vi "BRig_RT__Case_Exp__State_initTrial2.vi"(0 "input_dataCurrent":u16[](array[numeric]), 1 "input_dataTrial":u16[][](array[numeric]), 3 "input_dataExp":u16[](array[numeric]), 6 "input_dataBlock":u16[][](array[numeric]), 8 "input_dataLC":u16[](array[numeric])) -> (7 "output_L_Wrong_Laser_l2":bool, 9 "output_L_Wrong_Event_l2":bool, 10 "output_L_Power_l1":dbl, 11 "output_L_Reward_Laser_l2":bool, 12 "output_L_Power_l2":dbl, 13 "output_L_Reward_Event_l2":bool, 14 "output_dataCurrent":u16[](array[numeric]), 15 "output_dataTrial":u16[][](array[numeric]), 16 "output_L_Reward_Event_l1":bool, 17 "output_L_Reward_Laser_l1":bool, 18 "output_L_Wrong_Event_l1":bool, 19 "output_L_Wrong_Laser_l1":bool)   [LabVIEW 2014]
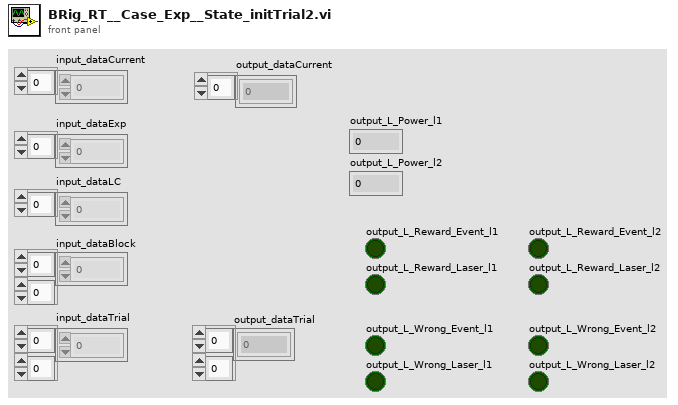
[diagram p1: front panel]
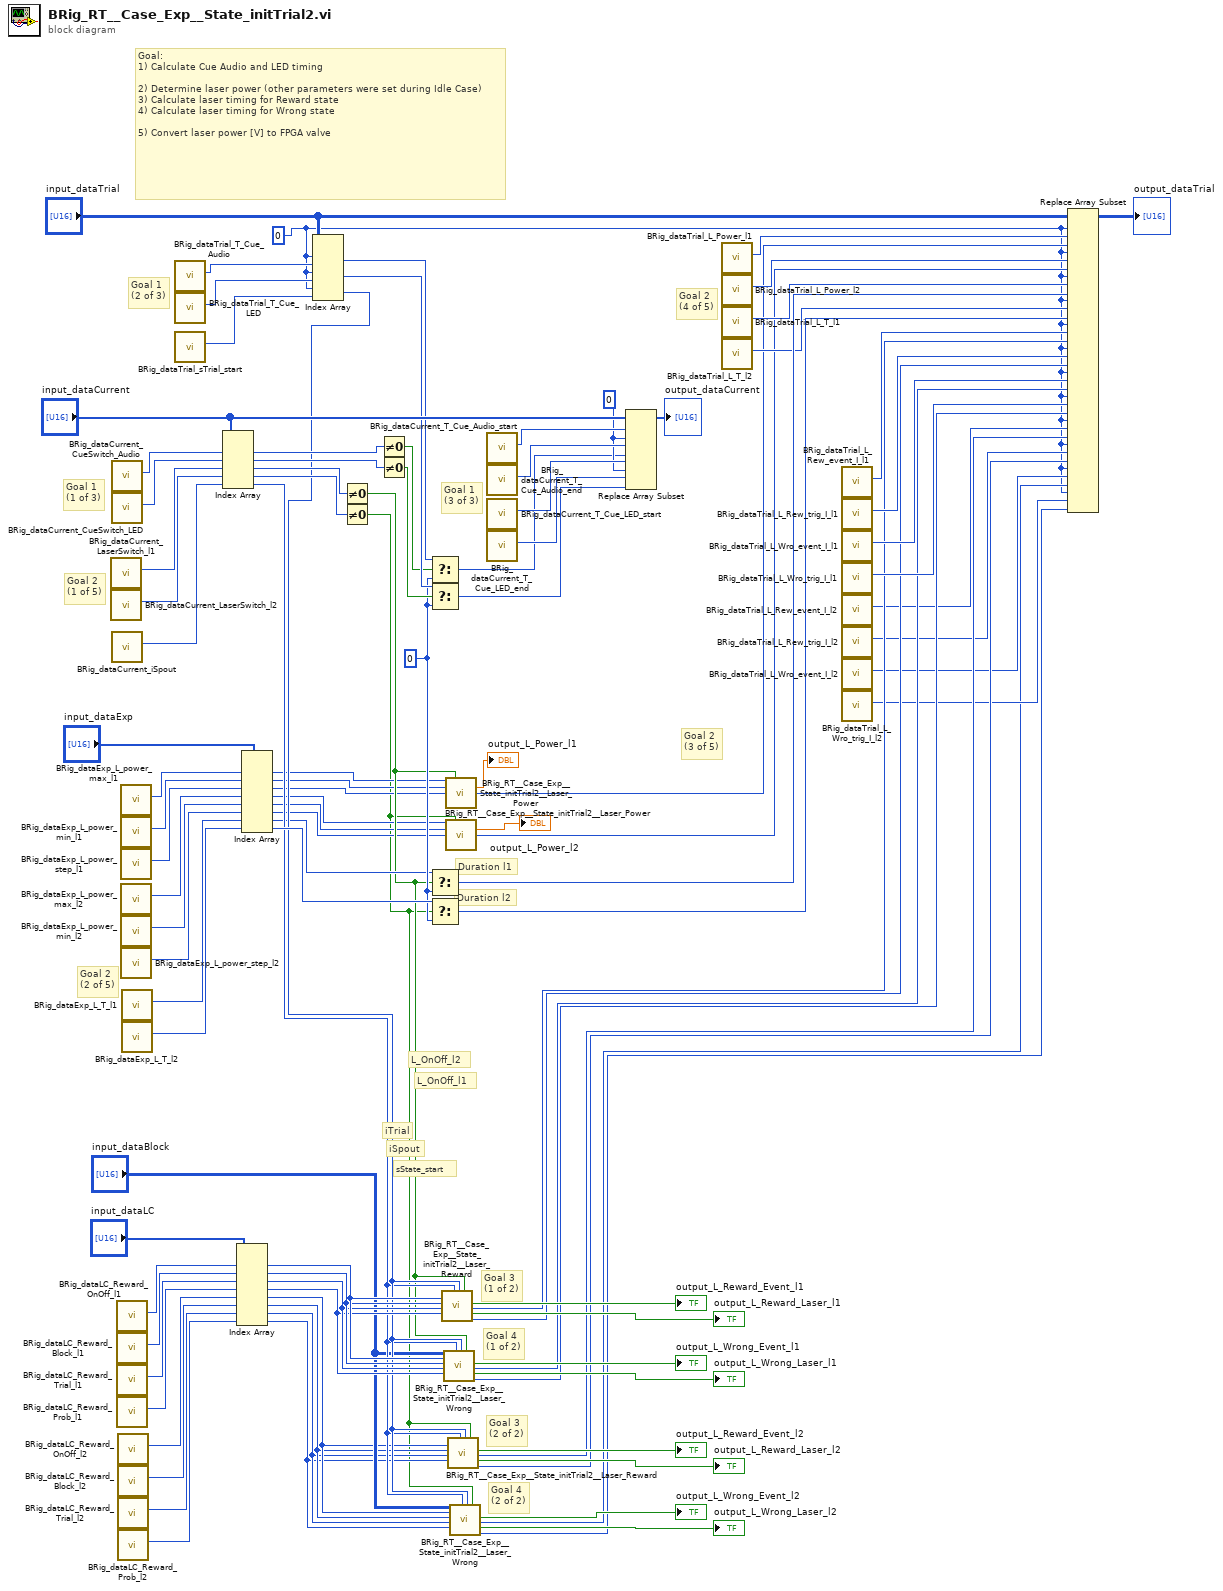
[diagram p0: block diagram]
diagram:
  w1 = 0
  w72 = u16 0 ("f")
  w93 = u16 0 ("new element/subarray")
  # "L_OnOff_l2"
  # "Goal 2\n(3 of 5)"
  # "Goal 4\n(2 of 2)"
  # "Goal 4\n(1 of 2)"
  # "Goal 3\n(2 of 2)"
  # "Goal 3\n(1 of 2)"
  # "L_OnOff_l1"
  # "iTrial"
  # "sState_start"
  # "iSpout"
  # "Goal 2\n(4 of 5)"
  # "Goal 2\n(2 of 5)"
  # "Duration l2"
  # "Duration l1"
  # "Goal 2\n(1 of 5)"
  # "Goal 1\n(3 of 3)"
  # "Goal 1\n(2 of 3)"
  # "Goal 1\n(1 of 3)"
  # "Goal:\n1) Calculate Cue Audio and LED timing\n\n2) Determine laser power (other parameters were set during Idle Case)\n3) Calculate laser timing for Reward state\n4) Calculate laser timing for Wrong state\n\n5) Convert laser power [V] to FPGA valve"
  n1 = call "BRig_dataCurrent_LaserSwitch_l1.vi"() -> ("output_LaserSwitch_l1"=w86:i32)  [unwired: 11 in]
  n2 = call "BRig_dataCurrent_LaserSwitch_l2.vi"() -> ("output_LaserSwitch_l2"=w85:i32)  [unwired: 11 in]
  n3 = call "BRig_dataCurrent_CueSwitch_Audio.vi"() -> ("output_CueSwitch_Audio"=w102:i32)  [unwired: 11 in]
  n4 = call "BRig_dataCurrent_CueSwitch_LED.vi"() -> ("output_CueSwitch_LED"=w100:i32)  [unwired: 11 in]
  n5 = call "BRig_dataCurrent_iSpout.vi"() -> ("output_iSpout"=w55:i32)  [unwired: 11 in]
  n6 = call "BRig_dataLC_Reward_OnOff_l1.vi"() -> ("output_Reward_OnOff"=w61:i32)  [unwired: 11 in]
  n7 = call "BRig_dataLC_Reward_Block_l1.vi"() -> ("output_Reward_Block"=w60:i32)  [unwired: 11 in]
  n8 = call "BRig_dataLC_Reward_Trial_l1.vi"() -> ("output_Reward_Trial"=w59:i32)  [unwired: 11 in]
  n9 = call "BRig_dataLC_Reward_Prob_l1.vi"() -> ("output_Reward_Prob"=w58:i32)  [unwired: 11 in]
  n10 = call "BRig_dataLC_Reward_OnOff_l2.vi"() -> ("output_Reward_OnOff_l2"=w49:i32)  [unwired: 11 in]
  n11 = call "BRig_dataLC_Reward_Block_l2.vi"() -> ("output_Reward_Block_l2"=w48:i32)  [unwired: 11 in]
  n12 = call "BRig_dataLC_Reward_Trial_l2.vi"() -> ("output_Reward_Trial_l2"=w47:i32)  [unwired: 11 in]
  n13 = call "BRig_dataLC_Reward_Prob_l2.vi"() -> ("output_Reward_Prob_l2"=w46:i32)  [unwired: 11 in]
  n14 = call "BRig_dataExp_L_power_max_l1.vi"() -> ("output_L_power_max_l1"=w83:i32)  [unwired: 11 in]
  n15 = call "BRig_dataExp_L_power_min_l1.vi"() -> ("output_L_power_min_l1"=w82:i32)  [unwired: 11 in]
  n16 = call "BRig_dataExp_L_power_step_l1.vi"() -> ("output_L_power_step_l1"=w81:i32)  [unwired: 11 in]
  n17 = call "BRig_dataExp_L_power_max_l2.vi"() -> ("output_L_power_max_l2"=w80:i32)  [unwired: 11 in]
  n18 = call "BRig_dataExp_L_power_min_l2.vi"() -> ("output_L_power_min_l2"=w79:i32)  [unwired: 11 in]
  n19 = call "BRig_dataExp_L_power_step_l2.vi"() -> ("output_L_power_step_l2"=w78:i32)  [unwired: 11 in]
  n20 = call "BRig_dataExp_L_T_l1.vi"() -> ("output_L_T_l1"=w77:i32)  [unwired: 11 in]
  n21 = call "BRig_dataExp_L_T_l2.vi"() -> ("output_L_T_l2"=w76:i32)  [unwired: 11 in]
  n22 = call "BRig_dataTrial_T_Cue_Audio.vi"() -> ("output_T_Cue_Audio"=w91:i32)  [unwired: 11 in]
  n23 = call "BRig_dataTrial_T_Cue_LED.vi"() -> ("output_T_Cue_LED"=w90:i32)  [unwired: 11 in]
  n24 = call "BRig_dataTrial_sTrial_start.vi"() -> ("output_sTrial_start"=w54:i32)  [unwired: 11 in]
  n25 = Index Array(array="input_dataCurrent", index #1=w102, index #2=w100, index #3=w86, index #4=w85, index #5=w55) -> (element #1=w95:u16, element #2=w94:u16, element #3=w57:u16, element #4=w56:u16, element #5=w44:u16)
  n26 = Index Array(array="input_dataLC", index #1=w61, index #2=w60, index #3=w59, index #4=w58, index #5=w49, index #6=w48, index #7=w47, index #8=w46) -> (element #1=w53:u16, element #2=w52:u16, element #3=w51:u16, element #4=w50:u16, element #5=w42:u16, element #6=w41:u16, element #7=w40:u16, element #8=w39:u16)
  n27 = Index Array(array="input_dataExp", index #1=w83, index #2=w82, index #3=w81, index #4=w80, index #5=w79, index #6=w78, index #7=w77, index #8=w76) -> (element #1=w12:u16, element #2=w11:u16, element #3=w10:u16, element #4=w7:u16, element #5=w6:u16, element #6=w5:u16, element #7=w14:u16, element #8=w73:u16)
  n28 = Index Array(array="input_dataTrial", index (row) #1=w1, index (col) #1=w91, index (row) #2=w1, index (col) #2=w90, index (row) #3=w1, index (col) #3=w54) -> (element #1=w89:u16, element #2=w88:u16, element #3=w45:u16)
  n29 = Not Equal To 0?(x=w57) -> (x != 0?=w13:bool)
  n30 = Not Equal To 0?(x=w56) -> (x != 0?=w4:bool)
  n31 = Not Equal To 0?(x=w95) -> (x != 0?=w75:bool)
  n32 = Not Equal To 0?(x=w94) -> (x != 0?=w74:bool)
  n33 = Select(t=w89, s=w75, f=w72) -> (s? t:f=w92:u16)
  n34 = Select(t=w88, s=w74, f=w72) -> (s? t:f=w87:u16)
  n35 = Select(t=w14, s=w13, f=w72) -> (s? t:f=w65:u16)
  n36 = Select(t=w73, s=w4, f=w72) -> (s? t:f=w63:u16)
  n37 = call "BRig_RT__Case_Exp__State_initTrial2__Laser_Reward.vi"("input_L_OnOff"=w53, "input_L_Block"=w52, "input_L_Trial"=w51, "input_L_Probability"=w50, "input_iSpout"=w44, "input_sState_start"=w45, "input_LaserSwitch"=w13) -> ("output_LR_Event"=→"output_L_Reward_Event_l1":bool, "output_LR_Event_num"=w26:u16, "output_LR_Laser"=→"output_L_Reward_Laser_l1":bool, "output_LR_Laser_num"=w25:u16)  [unwired: 9 in]
  n38 = call "BRig_RT__Case_Exp__State_initTrial2__Laser_Wrong.vi"("input_dataBlock"="input_dataBlock", "input_L_OnOff"=w53, "input_L_Block"=w52, "input_L_Trial"=w51, "input_L_Probability"=w50, "input_iSpout"=w44, "input_sState_start"=w45, "input_LaserSwitch"=w13) -> ("output_LR_Event"=→"output_L_Wrong_Event_l1":bool, "output_LR_Event_num"=w24:u16, "output_LR_Laser"=→"output_L_Wrong_Laser_l1":bool, "output_LR_Laser_num"=w23:u16)  [unwired: 8 in]
  n39 = call "BRig_RT__Case_Exp__State_initTrial2__Laser_Power.vi"("input_L_Power_max__x100"=w12, "input_LaserSwitch"=w13, "input_L_Power_min__x100"=w11, "input_L_Power_step__x100"=w10) -> ("output_L_Power"=→"output_L_Power_l1":dbl, "output_L_Power_x100"=w8:u16)  [unwired: 10 in]
  n40 = call "BRig_RT__Case_Exp__State_initTrial2__Laser_Power.vi"("input_L_Power_max__x100"=w7, "input_LaserSwitch"=w4, "input_L_Power_min__x100"=w6, "input_L_Power_step__x100"=w5) -> ("output_L_Power"=→"output_L_Power_l2":dbl, "output_L_Power_x100"=w2:u16)  [unwired: 10 in]
  n41 = call "BRig_RT__Case_Exp__State_initTrial2__Laser_Reward.vi"("input_L_OnOff"=w42, "input_L_Block"=w41, "input_L_Trial"=w40, "input_L_Probability"=w39, "input_iSpout"=w44, "input_sState_start"=w45, "input_LaserSwitch"=w4) -> ("output_LR_Event"=→"output_L_Reward_Event_l2":bool, "output_LR_Event_num"=w21:u16, "output_LR_Laser"=→"output_L_Reward_Laser_l2":bool, "output_LR_Laser_num"=w19:u16)  [unwired: 9 in]
  n42 = call "BRig_RT__Case_Exp__State_initTrial2__Laser_Wrong.vi"("input_dataBlock"="input_dataBlock", "input_L_OnOff"=w42, "input_L_Block"=w41, "input_L_Trial"=w40, "input_L_Probability"=w39, "input_iSpout"=w44, "input_sState_start"=w45, "input_LaserSwitch"=w4) -> ("output_LR_Event"=→"output_L_Wrong_Event_l2":bool, "output_LR_Event_num"=w16:u16, "output_LR_Laser"=→"output_L_Wrong_Laser_l2":bool, "output_LR_Laser_num"=w15:u16)  [unwired: 8 in]
  n43 = call "BRig_dataCurrent_T_Cue_Audio_start.vi"() -> ("output_T_Cue_Audio_start"=w99:i32)  [unwired: 11 in]
  n44 = call "BRig_dataCurrent_T_Cue_Audio_end.vi"() -> ("output_T_Cue_Audio_end"=w98:i32)  [unwired: 11 in]
  n45 = call "BRig_dataCurrent_T_Cue_LED_start.vi"() -> ("output_T_Cue_LED_start"=w97:i32)  [unwired: 11 in]
  n46 = call "BRig_dataCurrent_T_Cue_LED_end.vi"() -> ("output_T_Cue_LED_end"=w96:i32)  [unwired: 11 in]
  n47 = Replace Array Subset(array="input_dataCurrent", new element #1=w93, index #1=w99, new element #2=w92, index #2=w98, new element #3=w93, index #3=w97, new element #4=w87, index #4=w96) -> (→"output_dataCurrent":u16[])
  n48 = call "BRig_dataTrial_L_Power_l1.vi"() -> ("output_L_Power_l1"=w68:i32)  [unwired: 11 in]
  n49 = call "BRig_dataTrial_L_Power_l2.vi"() -> ("output_L_Power_l2"=w67:i32)  [unwired: 11 in]
  n50 = call "BRig_dataTrial_L_T_l1.vi"() -> ("output_L_T_l1"=w66:i32)  [unwired: 11 in]
  n51 = call "BRig_dataTrial_L_T_l2.vi"() -> ("output_L_T_l2"=w64:i32)  [unwired: 11 in]
  n52 = call "BRig_dataTrial_L_Rew_event_I_l1.vi"() -> ("output_L_Rew_event_I_l1"=w34:i32)  [unwired: 11 in]
  n53 = call "BRig_dataTrial_L_Rew_trig_I_l1.vi"() -> ("output_L_Rew_trig_I_l1"=w33:i32)  [unwired: 11 in]
  n54 = call "BRig_dataTrial_L_Wro_event_I_l1.vi"() -> ("output_L_Wro_event_I_l1"=w32:i32)  [unwired: 11 in]
  n55 = call "BRig_dataTrial_L_Wro_trig_I_l1.vi"() -> ("output_L_Wro_trig_I_l1"=w31:i32)  [unwired: 11 in]
  n56 = call "BRig_dataTrial_L_Rew_event_I_l2.vi"() -> ("output_L_Rew_event_I_l2"=w22:i32)  [unwired: 11 in]
  n57 = call "BRig_dataTrial_L_Rew_trig_I_l2.vi"() -> ("output_L_Rew_trig_I_l2"=w20:i32)  [unwired: 11 in]
  n58 = call "BRig_dataTrial_L_Wro_event_I_l2.vi"() -> ("output_L_Wro_event_I_l2"=w18:i32)  [unwired: 11 in]
  n59 = call "BRig_dataTrial_L_Wro_trig_I_l2.vi"() -> ("output_L_Wro_trig_I_l2"=w17:i32)  [unwired: 11 in]
  n60 = Replace Array Subset(array="input_dataTrial", new element #1=w8, index (row) #1=w1, index (col) #1=w68, new element #2=w2, index (row) #2=w1, index (col) #2=w67, new element #3=w65, index (row) #3=w1, index (col) #3=w66, new element #4=w63, index (row) #4=w1, index (col) #4=w64, new element #5=w26, index (row) #5=w1, index (col) #5=w34, new element #6=w25, index (row) #6=w1, index (col) #6=w33, new element #7=w24, index (row) #7=w1, index (col) #7=w32, new element #8=w23, index (row) #8=w1, index (col) #8=w31, new element #9=w21, index (row) #9=w1, index (col) #9=w22, new element #10=w19, index (row) #10=w1, index (col) #10=w20, new element #11=w16, index (row) #11=w1, index (col) #11=w18, new element #12=w15, index (row) #12=w1, index (col) #12=w17) -> (→"output_dataTrial":u16[][])
